vi "SPC_get_mode.vi"(8 "Error In":errorcluster, 11 "DLL Path":path) -> (0 "Error Out":errorcluster, 1 "Current Mode Value":i16, 2 "Explanation":string, 3 "DLL Path":path)   [LabVIEW 2017]
doc: "The procedure returns the current DLL operation mode. Possible ‘mode’ values are defined in the spcm_def.h file:\n#define SPC_HARD 0 /* hardware mode */\n#define SPC_SIMUL600 600 /* simulation mode of SPC600 module */\n#define SPC_SIMUL630 630 /* simulation mode of SPC630 module */\n#define SPC_SIMUL700 700 /* simulation mode of SPC700 module */\n#define SPC_SIMUL730 730 /* simulation mode of SPC730 module */\n#define SPC_SIMUL130 130 /* simulation mode of SPC130 module */\n#define SPC_SIMUL830 830 /* simulation mode of SPC830 module */\n#define SPC_SIMUL140 140 /* simulation mode of SPC140 module */\n#define SPC_SIMUL930 930 /* simulation mode of SPC930 module */\n#define SPC_SIMUL150 150 /* simulation mode of SPC150 module */\n#define DPC_SIMUL230 230 /* simulation mode of DPC230 module */\n#define SPC_SIMUL131 131 /* simulation mode of SPC131 ( = SPC-130-EM) module */\n#define SPC_SIMUL151 151 /* simulation mode of SPC150N module */\n#define SPC_SIMUL160 160 /* simulation mode of SPC160 module */\n\ninfo@becker-hickl.de"
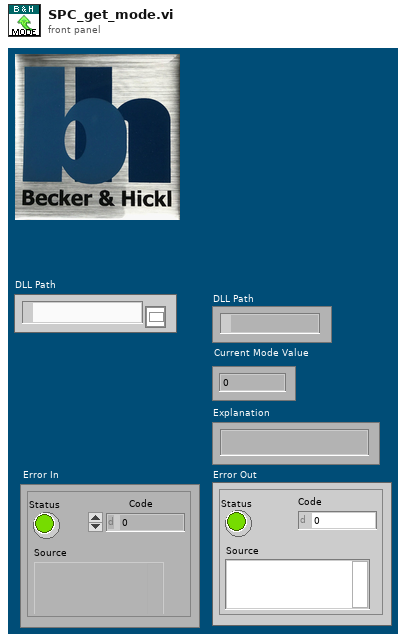
[diagram p1: front panel]
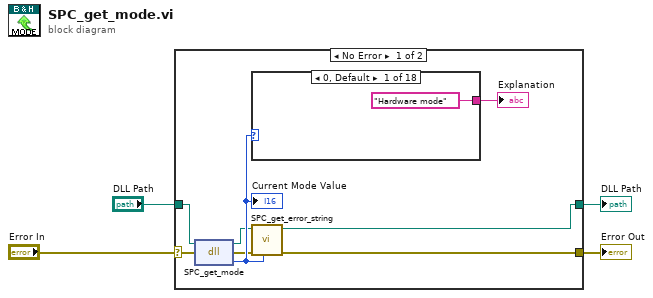
[diagram p0: block diagram]
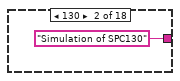
[diagram p2: hidden frame]
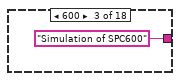
[diagram p3: hidden frame]
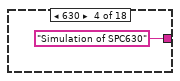
[diagram p4: hidden frame]
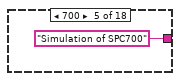
[diagram p5: hidden frame]
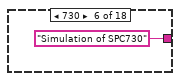
[diagram p6: hidden frame]
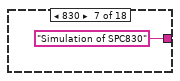
[diagram p7: hidden frame]
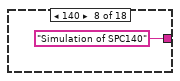
[diagram p8: hidden frame]
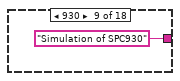
[diagram p9: hidden frame]
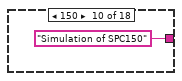
[diagram p10: hidden frame]
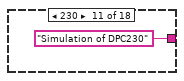
[diagram p11: hidden frame]
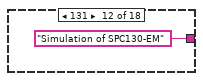
[diagram p12: hidden frame]
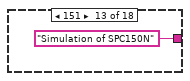
[diagram p13: hidden frame]
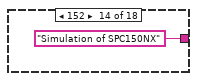
[diagram p14: hidden frame]
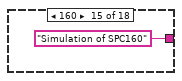
[diagram p15: hidden frame]
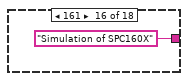
[diagram p16: hidden frame]
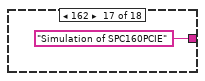
[diagram p17: hidden frame]
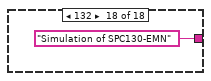
[diagram p18: hidden frame]
diagram:
  n1 = case shown="No Error" "Error In" {
    selector: "Error In" -> [w10 w31]
    tunnel: "DLL Path" -> [w11 w32]
    tunnel: [w6 w32] -> w3
    tunnel: [w7 w31] -> w2
    frame No Error {
      n2 = dll-call lib="D:/spcm/lib/lab_view/lv10.0/spcm32.dll" fn="SPC_get_mode"(path in=w11, error in=w10) -> (path out=w5:path, error out=w8:errorcluster, "return type"=w9:i16)  [unwired: 1 in]
      "Current Mode Value" <- w9
      n3 = case shown="0, Default" w9 {
        tunnel: ["Hardware mode" "Simulation of SPC130" "Simulation of SPC600" "Simulation of SPC630" "Simulation of SPC700" "Simulation of SPC730" "Simulation of SPC830" "Simulation of SPC140" "Simulation of SPC930" "Simulation of SPC150" "Simulation of DPC230" "Simulation of SPC130-EM" "Simulation of SPC150N" "Simulation of SPC150NX" "Simulation of SPC160" "Simulation of SPC160X" "Simulation of SPC160PCIE" "Simulation of SPC130-EMN"] -> w12
        frame 0, Default {
        }
        frame 130 {
        }
        frame 600 {
        }
        frame 630 {
        }
        frame 700 {
        }
        frame 730 {
        }
        frame 830 {
        }
        frame 140 {
        }
        frame 930 {
        }
        frame 150 {
        }
        frame 230 {
        }
        frame 131 {
        }
        frame 151 {
        }
        frame 152 {
        }
        frame 160 {
        }
        frame 161 {
        }
        frame 162 {
        }
        frame 132 {
        }
      }
      "Explanation" <- w12
      n4 = call "SPC_get_error_string.vi"("ErrorID"=w9, "Error In"=w8, "DLL Path"=w5) -> ("Error Out"=w7:errorcluster, "DLL Path"=w6:path)  [unwired: 6 in, 1 out]
    }
    frame Error {
    }
  }
  "DLL Path" <- w3
  "Error Out" <- w2
